vi "Border Offset.vi"() -> (3 "Border Offset (px)":i32=10)   [LabVIEW 2014]
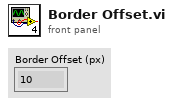
[diagram p1: front panel]
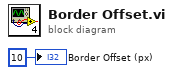
[diagram p0: block diagram]
diagram:
  "Border Offset (px)" <- 10
